vi "ToPythonVersionString.vi"(11 "python version":T1) -> (3 "python version string":string)   [LabVIEW 2020]
doc: "Helper VI to convert from the Python version enum to a version string that is the input to the Open Python Session node."
uses:
  PythonVersionsEnum.ctl
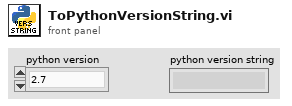
[diagram p1: front panel]
types:
  T1 = typedef "PythonVersionsEnum.ctl" = enum16{"2.7", "3.6"}
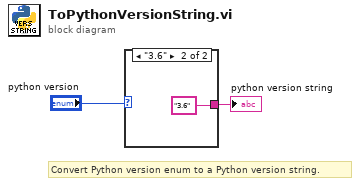
[diagram p0: block diagram]
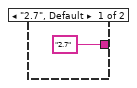
[diagram p2: hidden frame]
diagram:
  # "Convert Python version enum to a Python version string."
  n1 = case shown="\"3.6\"" "python version" {
    tunnel: ["2.7" ("python version") "3.6" ("python version")] -> w1
    frame "2.7", Default {
    }
    frame "3.6" {
    }
  }
  "python version string" <- w1
